vi "Align Block.vi"(10 "Command":enum16{"distance", "align", "rotate"}(ring), 11 "Camera In":T4) -> (1 "Block in front?":bool, 3 "Robot Velocities":T1)   [LabVIEW 2012]
uses:
  Globals.vi
  <vilib>/vision/Image Controls.llb/IMAQ Image.ctl
  <vilib>/httpClient/ClientHandle.ctl
  <vilib>/httpClient/LabVIEWHTTPClient.lvlib
panel:
  out "Block aligned?":bool
  out "Block centered?":bool
  in  "Arc radius":dbl=0.3
  in  "Rotate speed (rad/s)":dbl=0.3
  in  "Angle deadband":dbl=5.0
  in  "strafe velocity":dbl
  in  "Safe distance sides":dbl
  in  "Forward Speed":dbl
  in  "Safe distance":dbl
  in  "Block range":dbl
  in  "Block deadband":dbl
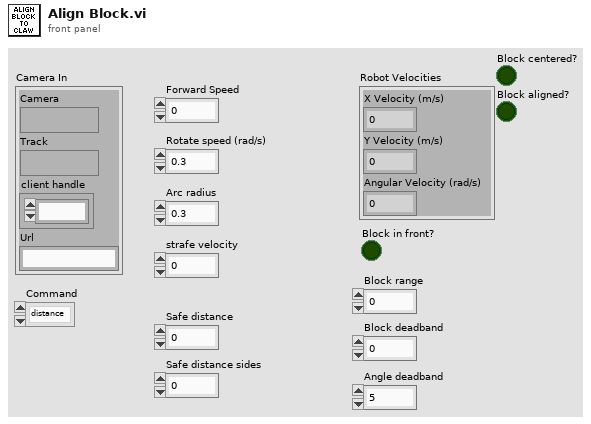
[diagram p1: front panel]
types:
  T1 = cluster{"X Velocity (m/s)":dbl, "Y Velocity (m/s)":dbl, "Angular Velocity (rad/s)":dbl}
  T2 = typedef "IMAQ Image.ctl" = refnum<image>
  T3 = typedef "LabVIEWHTTPClient.lvlib/ClientHandle.ctl" = refnum<k1>
  T4 = cluster{"Camera":T2, "Track":T2, "client handle":T3, "Url":string}
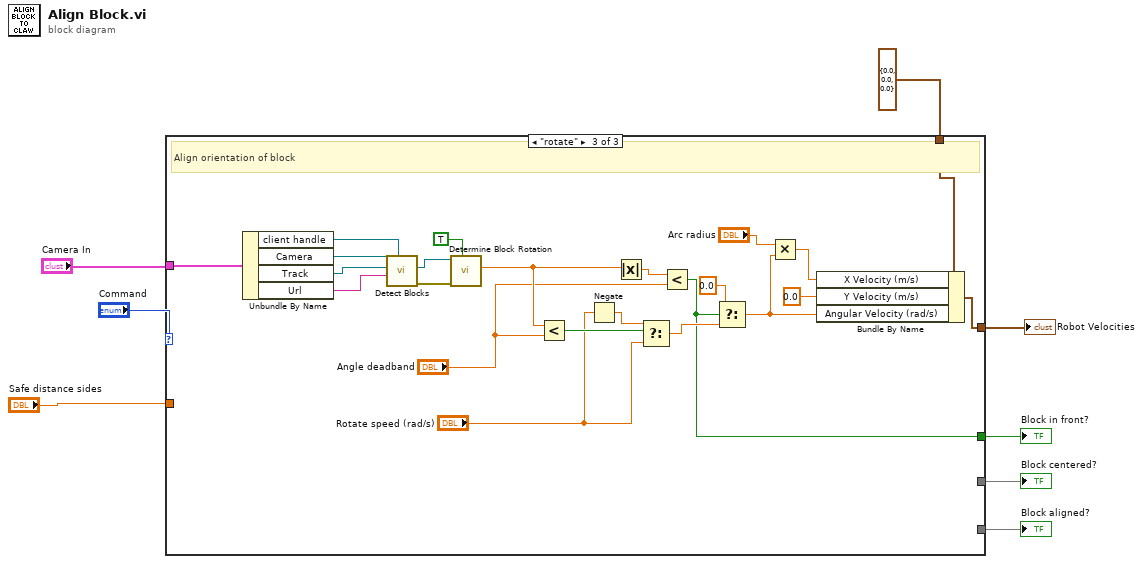
[diagram p0: block diagram]
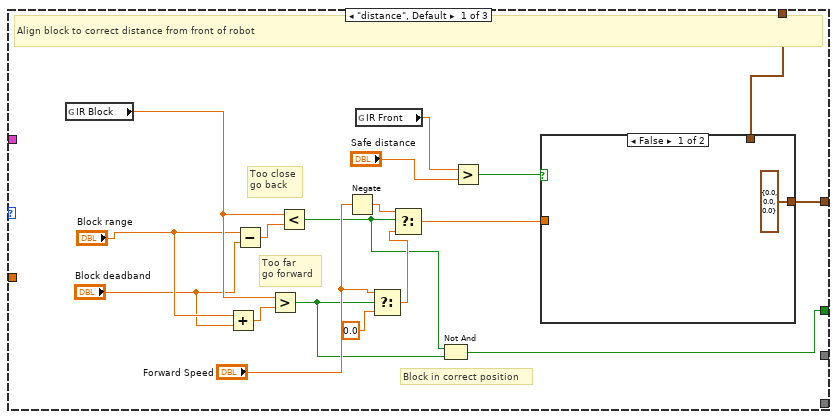
[diagram p2: hidden frame]
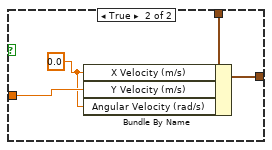
[diagram p3: hidden frame]
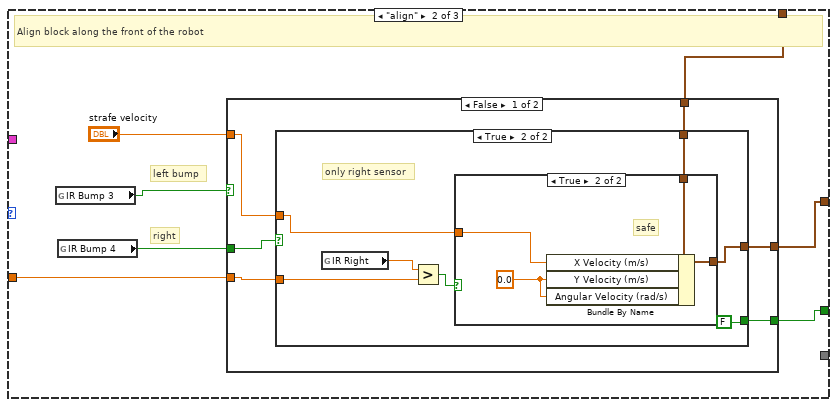
[diagram p4: hidden frame]
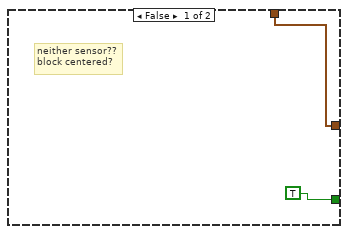
[diagram p5: hidden frame]
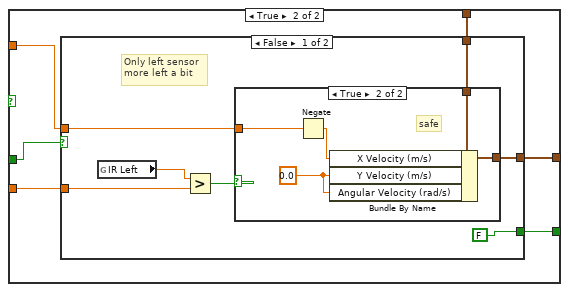
[diagram p7: hidden frame]
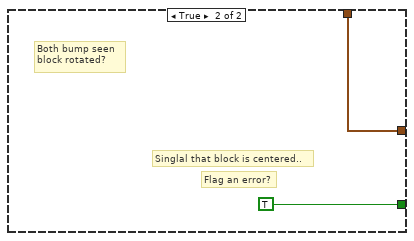
[diagram p9: hidden frame]
diagram:
  n1 = case shown="\"rotate\"" "Command" {
    tunnel: T1 {"X Velocity (m/s)"=0.0, "Y Velocity (m/s)"=0.0, "Angular Velocity (rad/s)"=0.0} ("Robot Velocities") -> [w11 w35 w85]
    tunnel: [w10 w36 w84] -> w6
    tunnel: [w9 w34 w86] -> w5
    tunnel: "Camera In" -> [_ _ w90]
    tunnel: "Safe distance sides" -> [_ w33 _]
    tunnel: [_ _ _] -> w2
    tunnel: [_ _ _] -> w1
    frame "distance", Default {
      # "Block in correct position"
      # "Too far\ngo forward"
      # "Too close\ngo back"
      # "Align block to correct distance from front of robot"
      n2 = global read "Globals.vi" "IR Block"() -> (w25:dbl)
      n3 = Add(x="Block range", y="Block deadband") -> (x+y=w24:dbl)
      n4 = Subtract(x="Block range", y="Block deadband") -> (x-y=w26:dbl)
      n5 = Greater?(x=w25, y=w24) -> (0:w12:bool)
      n6 = Less?(x=w25, y=w26) -> (x < y?=w13:bool)
      n7 = Negate(x="Forward Speed") -> (-x=w17:dbl)
      n8 = global read "Globals.vi" "IR Front"() -> (w21:dbl)
      n9 = Select(t="Forward Speed", s=w12, f=0.0) -> (s? t:f=w18:dbl)
      n10 = Select(t=w17, s=w13, f=w18) -> (s? t:f=w14:dbl)
      n11 = Not And(1:w12, 2:w13) -> (0:w9:bool)
      n12 = Greater?(x=w21, y="Safe distance") -> (0:w19:bool)
      n13 = case shown="False" w19 {
        tunnel: w14 -> [_ w29]
        tunnel: w11 -> [_ w31]
        tunnel: [T1 {"X Velocity (m/s)"=0.0, "Y Velocity (m/s)"=0.0, "Angular Velocity (rad/s)"=0.0} ("Robot Velocities") w30] -> w10
        frame False {
        }
        frame True {
          w28 = 0.0 ("X Velocity (m/s)")
          n14 = Bundle By Name(cluster=w31, "X Velocity (m/s)"=w28, "Y Velocity (m/s)"=w29, "Angular Velocity (rad/s)"=w28) -> (w30:T1)
        }
      }
    }
    frame "align" {
      # "right"
      # "left bump"
      # "Align block along the front of the robot"
      n15 = global read "Globals.vi" "IR Bump 3"() -> (w38:bool)
      n16 = global read "Globals.vi" "IR Bump 4"() -> (w37:bool)
      n17 = case shown="False" w38 {
        tunnel: w37 -> [w44 w64]
        tunnel: [w42 w63] -> w36
        tunnel: w35 -> [w43 w62]
        tunnel: [w41 w61] -> w34
        tunnel: w33 -> [w40 w60]
        tunnel: "strafe velocity" -> [w39 w59]
        frame False {
          n18 = case shown="True" w44 {
            tunnel: w43 -> [w46 w51]
            tunnel: [w46 w50] -> w42
            tunnel: [TRUE FALSE] -> w41
            tunnel: w40 -> [_ w48]
            tunnel: w39 -> [_ w47]
            frame False {
              # "neither sensor??\nblock centered?"
            }
            frame True {
              # "only right sensor"
              n19 = global read "Globals.vi" "IR Right"() -> (w53:dbl)
              n20 = Greater?(x=w53, y=w48) -> (0:w52:bool)
              n21 = case shown="True" w52 {
                tunnel: [w54 w57] -> w50
                tunnel: w51 -> [w54 w58]
                tunnel: w47 -> [_ w55]
                frame False {
                  # "panic!"
                }
                frame True {
                  w56 = 0.0 ("Y Velocity (m/s)")
                  # "safe"
                  n22 = Bundle By Name(cluster=w58, "X Velocity (m/s)"=w55, "Y Velocity (m/s)"=w56, "Angular Velocity (rad/s)"=w56) -> (w57:T1)
                }
              }
            }
          }
        }
        frame True {
          n23 = case shown="False" w64 {
            tunnel: [w69 w78] -> w63
            tunnel: w62 -> [w68 w78]
            tunnel: [FALSE TRUE] -> w61
            tunnel: w60 -> [w66 _]
            tunnel: w59 -> [w65 _]
            frame False {
              # "Only left sensor\nmore left a bit"
              n24 = global read "Globals.vi" "IR Left"() -> (w71:dbl)
              n25 = Greater?(x=w71, y=w66) -> (0:w70:bool)
              n26 = case shown="True" w70 {
                tunnel: [w72 w76] -> w69
                tunnel: w68 -> [w72 w77]
                tunnel: w65 -> [_ w73]
                frame False {
                  # "panic!"
                }
                frame True {
                  w74 = 0.0 ("Y Velocity (m/s)")
                  # "safe"
                  n27 = Negate(x=w73) -> (-x=w75:dbl)
                  n28 = Bundle By Name(cluster=w77, "X Velocity (m/s)"=w75, "Y Velocity (m/s)"=w74, "Angular Velocity (rad/s)"=w74) -> (w76:T1)
                }
              }
            }
            frame True {
              # "Flag an error?"
              # "Singlal that block is centered.."
              # "Both bump seen\nblock rotated?"
            }
          }
        }
      }
    }
    frame "rotate" {
      # "Align orientation of block"
      n29 = Unbundle By Name(w90) -> ("client handle"=w100:T3, "Camera"=w101:T2, "Track"=w102:T2, "Url"=w97:string)
      n30 = call "Detect Blocks.vi"("client handle"=w100, "Url"=w97, "Image Dst"=w102, "Refnum in"=w101) -> ("error out"=w98:errorcluster, "Detected Image Out"=w99:T2)  [unwired: 5 in, 1 out]
      n31 = call "Determine Block Rotation.vi"("Show line?"=TRUE, "error in (no error)"=w98, "Image in"=w99) -> ("Angle (Pixel)"=w96:dbl)  [unwired: 5 in, 3 out]
      n32 = Less?(x=w96, y="Angle deadband") -> (x < y?=w94:bool)
      n33 = Negate(x="Rotate speed (rad/s)") -> (-x=w88:dbl)
      n34 = Absolute Value(x=w96) -> (abs(x)=w95:dbl)
      n35 = Select(t=w88, s=w94, f="Rotate speed (rad/s)") -> (s? t:f=w93:dbl)
      n36 = Less?(x=w95, y="Angle deadband") -> (x < y?=w86:bool)
      n37 = Select(t=0.0, s=w86, f=w93) -> (s? t:f=w82:dbl)
      n38 = Multiply(x="Arc radius", y=w82) -> (x*y=w81:dbl)
      n39 = Bundle By Name(cluster=w85, "X Velocity (m/s)"=w81, "Y Velocity (m/s)"=0.0, "Angular Velocity (rad/s)"=w82) -> (w84:T1)
    }
  }
  "Robot Velocities" <- w6
  "Block in front?" <- w5
  "Block centered?" <- w1
  "Block aligned?" <- w2
